vi "Prepend.vi"(2 "bytestream":refnum<class "Bytestream.lvclass">, 3 "x":u8[](array[numeric]) format="%02x") -> (0 "bytestream out":refnum<class "Bytestream.lvclass">)   [LabVIEW 2020, in "NI_Bytestream.lvlib" / "Bytestream.lvclass"]
uses:
  <vilib>/Array/Bytestream/Bytestream.lvclass
  <vilib>/Array/Bytestream/Bytestream.lvclass/Bytestream.ctl
  <vilib>/Array/Bytestream/Datum.ctl
  <vilib>/Array/Bytestream/Count Allocated Datums.vi
  <vilib>/Array/Bytestream/Count Datums.vi
  <vilib>/Array/Bytestream/Grow Datum Array.vi
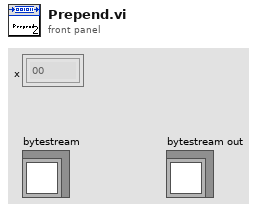
[diagram p1: front panel]
types:
  T1 = typedef "NI_Bytestream.lvlib/Bytestream.lvclass/Datum.ctl" = cluster{"array":u8[], "index":i32}
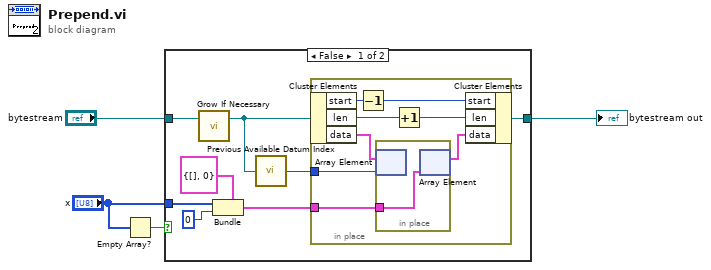
[diagram p0: block diagram]
diagram:
  n1 = Empty Array?(array="x") -> (empty?=w2:bool)
  n2 = case shown="False" w2 {
    tunnel: "bytestream" -> [w8 w22]
    tunnel: [w12 w22] -> w1
    tunnel: "x" -> [w11 _]
    frame False {
      n3 = call <vilib>:"Grow If Necessary.vi"("bytestream in"=w8) -> ("bytestream out"=w6:refnum<class "Bytestream.lvclass">)  [unwired: 2 in]
      n4 = Bundle(cluster=T1 {"array"=[], "index"=0} ("datum"), "array"=w11, "index"=0) -> (w9:T1)
      n5 = call <vilib>:"Previous Available Datum Index.vi"("bytestream"=w6) -> ("index"=w5:i32)
      n6 = in-place {
        in-place-border: w9 -> [w18]
        in-place-border: w5 -> [w19]
        n7 = in-place-cluster #1(w6) -> ("start"=w14:i32, "len"=w16:i32, "data"=w20:T1[])
        n8 = Decrement(x=w14) -> (x-1=w13:i32)
        n9 = in-place {
          in-place-border: w18 -> [w21]
          n10 = in-place-array #2(w20, w19) -> ()  [unwired: 1 out]
          n11 = in-place-array #2(w21) -> (w17:T1[])  [unwired: 1 out]
        }
        n12 = Increment(x=w16) -> (x+1=w15:i32)
        n13 = in-place-cluster #1("start"=w13, "len"=w15, "data"=w17) -> (w12:refnum<class "Bytestream.lvclass">)
      }
    }
    frame True {
    }
  }
  "bytestream out" <- w1
